vi "hwOperation_hwDisconnect.vi"(7 "hwType":string, 8 "error in":errorcluster, 11 "hwDriverRef in":T1) -> (0 "error out":errorcluster, 3 "hwDriverRef out":T1)   [LabVIEW 2016]
uses:
  QX/hw_QX_hwDriverRef.ctl
  C:/Users/CL/Desktop/ZcDAQprj0811/ZcDAQprj/Modules/DAQ-Device/Hardware Drivers/QX/HBM LabVIEW Driver/DLLs/Hbm.Api.Common.dll
  QX/HBM LabVIEW Driver/DLLs/Hbm.Api.Common.dll
  C:/Users/CL/Desktop/ZcDAQprj0811/ZcDAQprj/Modules/DAQ-Device/Hardware Drivers/QX/HBM LabVIEW Driver/DLLs/Hbm.Api.LabVIEW.dll
  QX/HBM LabVIEW Driver/DLLs/Hbm.Api.LabVIEW.dll
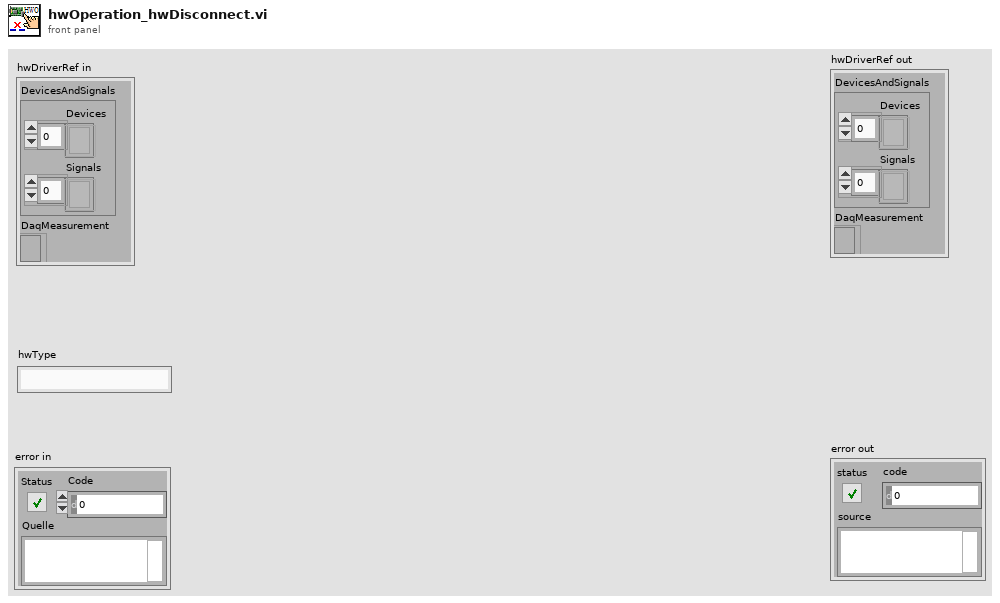
[diagram p1: front panel]
types:
  T1 = typedef "hw_QX_hwDriverRef.ctl" = cluster{"DevicesAndSignals":cluster{"Devices":refnum<k24>[], "Signals":refnum<k24>[]}, "DaqMeasurement":refnum<k24>}
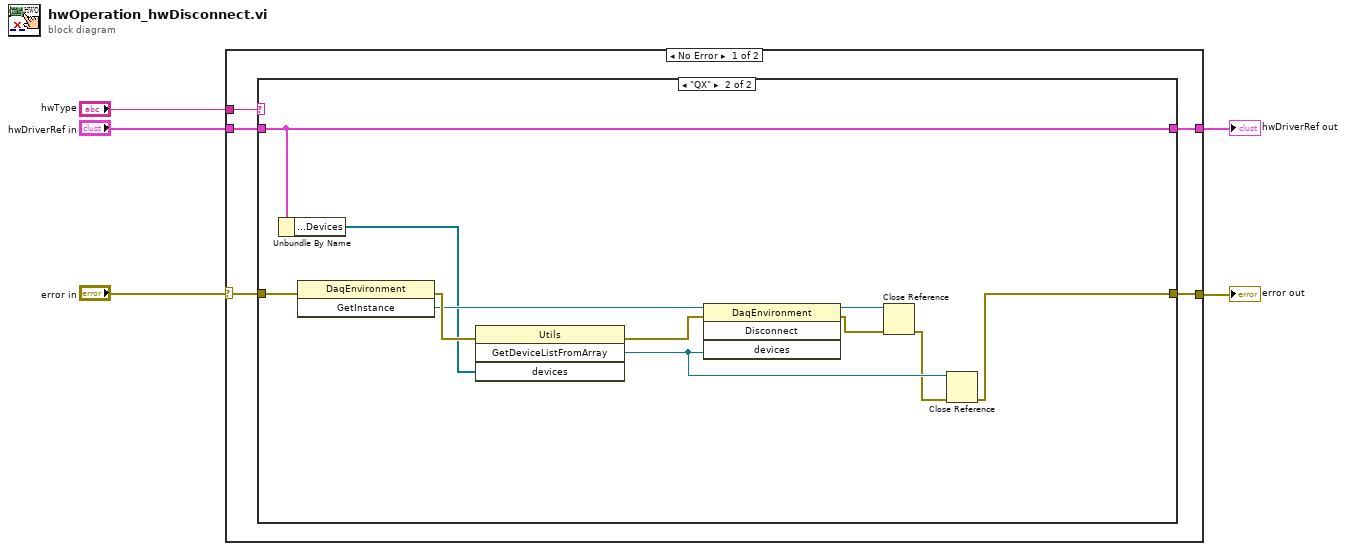
[diagram p0: block diagram]
diagram:
  n1 = case shown="No Error" "error in" {
    selector: "error in" -> [w9 w25]
    tunnel: [w10 w25] -> w4
    tunnel: "hwType" -> [w8 _]
    tunnel: "hwDriverRef in" -> [w7 w24]
    tunnel: [w6 w24] -> w1
    frame No Error {
      n2 = case shown="\"QX\"" w8 {
        tunnel: [w12 w13] -> w10
        tunnel: w9 -> [w12 w14]
        tunnel: w7 -> [w11 w16]
        tunnel: [w11 w16] -> w6
        frame "Simulation", Default {
        }
        frame "QX" {
          n3 = Unbundle By Name(w16) -> ("DevicesAndSignals.Devices"=w15:refnum<k24>[])
          n4 = invoke on="Methodenknoten" class="DaqEnvironment" method="GetInstance"(error in=w14) -> (error out=w19:errorcluster, "GetInstance"=w18:refnum<k24>)  [unwired: 2 in, 1 out]
          n5 = invoke on="Methodenknoten" class="Utils" method="GetDeviceListFromArray"(error in=w19, "devices"=w15) -> (error out=w17:errorcluster, "GetDeviceListFromArray"=w23:refnum<k24>)  [unwired: 2 in, 2 out]
          n6 = invoke class="DaqEnvironment" method="Disconnect"(reference=w18, error in=w17, "devices"=w23) -> (reference out=w21:refnum<k24>, error out=w20:errorcluster)  [unwired: 1 in, 2 out]
          n7 = Close Reference(reference=w21, error in (no error)=w20) -> (error out=w22:errorcluster)
          n8 = Close Reference(reference=w23, error in (no error)=w22) -> (error out=w13:errorcluster)
        }
      }
    }
    frame Error {
    }
  }
  "error out" <- w4
  "hwDriverRef out" <- w1
